vi "Get Controls Indicators Status by name.vi"(7 "Enable (T)/Disable&GrayOut (F)":bool, 8 "error in (no error)":errorcluster, 11 "aray of references":refnum<vi>[](array[refnum])) -> (0 "error out":errorcluster, 3 "Status description":string)   [LabVIEW 2020, in "ATM.lvlib"]
doc: "This vi is meant to show if the objects in the FP have been disabled&greyout or enabled"
uses:
  ATM.lvlib
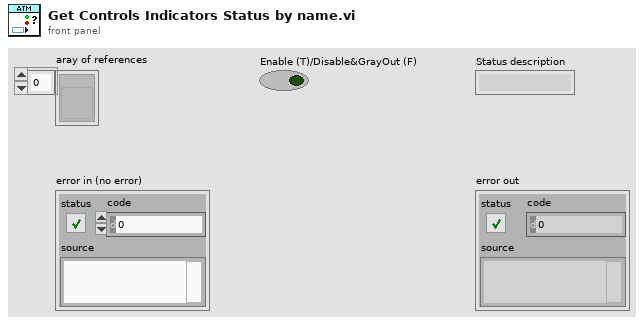
[diagram p1: front panel]
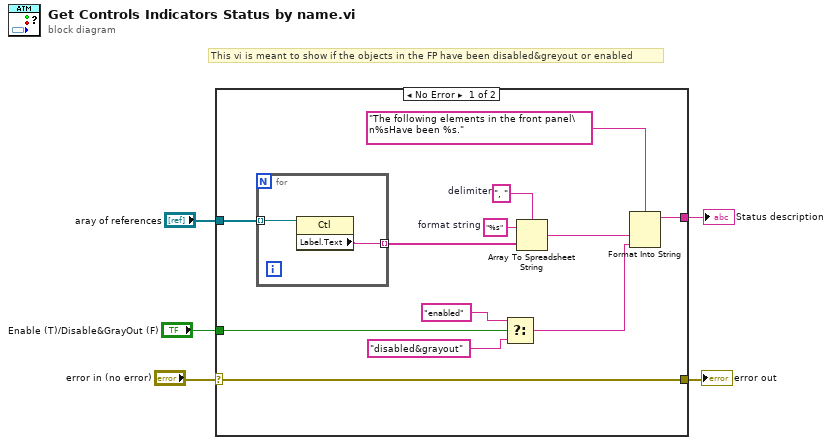
[diagram p0: block diagram]
diagram:
  # "This vi is meant to show if the objects in the FP have been disabled&greyout or enabled"
  n1 = case shown="No Error" "error in (no error)" {
    selector: "error in (no error)" -> [w6 w20]
    tunnel: "aray of references" -> [w17 _]
    tunnel: "Enable (T)/Disable&GrayOut (F)" -> [w9 _]
    tunnel: [w7 _] -> w3
    tunnel: [w6 w20] -> w2
    frame No Error {
      w14 = "%s"  # format string
      w15 = ", "  # delimiter
      n2 = for {
        tunnel: w17 -> [w19] mode=indexing
        tunnel: [w18] -> w16 mode=indexing
        n3 = property class="Ctl"(reference=w19) -> ("Label.Text"=w18:string)  [unwired: 1 in, 2 out]
      }
      n4 = Select(t="enabled" ("format string"), s=w9, f="disabled&grayout" ("format string")) -> (s? t:f=w8:string)
      n5 = Array To Spreadsheet String(delimiter (Tab)=w15, array=w16, 3:w14) -> (spreadsheet string=w12:string)
      n6 = Format Into String(format string="The following elements in the front panel\n%sHave been %s.", w12, w8) -> (resulting string=w7:string)  [unwired: 2 in, 1 out]
    }
    frame Error {
    }
  }
  "Status description" <- w3
  "error out" <- w2
